vi "Pause.vi"(8 "Tone (440 Hz)":u16=250, 9 "Line":i16(ring) items=["1", "2", "3", "4", "5", "6", "7", "8"], 10 "Text":string, 11 "NXT":T1) -> (3 "NXT 2":T1 caption="NXT")   [LabVIEW 2012]
uses:
  <vilib>/NXT/Subs/LVHSConnector.ctl
  <vilib>/NXT/LegoClasses/BrickReference/BrickReference.lvclass
  <vilib>/NXT/Block Support/NXT_ButtonSelector.ctl
  <vilib>/NXT/Dual Mode Library/Sound/Tone.vi
  <vilib>/NXT/Dual Mode Library/Display/drawText.vi
  <vilib>/NXT/Dual Mode Library/Sensors/readNXTButton.vi
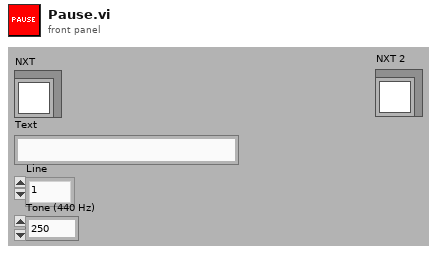
[diagram p1: front panel]
types:
  T1 = typedef "LVHSConnector.ctl" = refnum<class "BrickReference.lvclass">
  T2 = typedef "NXT_ButtonSelector.ctl" = u16
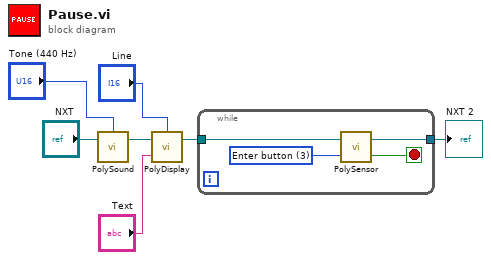
[diagram p0: block diagram]
diagram:
  n1 = call-poly <vilib>:"PolySound.vi"("NXT"="NXT", "Tone (440 Hz)"="Tone (440 Hz)") -> ("NXT"=w5:T1)  [unwired: 2 in]
  n2 = call-poly <vilib>:"PolyDisplay.vi"("Text"="Text", "NXT"=w5, "Line"="Line") -> ("NXT"=w4:T1)  [unwired: 1 in]
  n3 = while {
    tunnel: [w9] -> w6
    tunnel: w4 -> [w8]
    stop <- w10 stop-if-true
    w11 = T2 3 items=["Enter button"=3, "Left button"=2, "Right button"=1] ("Button (Enter button)")
    n4 = call-poly <vilib>:"PolySensor.vi"("Button (Enter button)"=w11, "NXT"=w8) -> ("Yes/No"=w10:bool, "NXT"=w9:T1)  [unwired: 1 in]
  }
  "NXT 2" <- w6
